vi "fpga_Ref Filter (60Hz).vi"(7 "reset":bool, 9 "input valid":bool, 11 "input data":fxp<+/-,24,1>) -> (1 "output valid":bool, 3 "output data <i24,3>":fxp<+/-,24,3> format="%.22g", 4 "ready for input":bool)   [LabVIEW 2011, in "NI_EP_Resample_FPGA.lvlib"]
uses:
  <vilib>/addons/Electrical Power/PQ/Resampling/NI_EP_Resample_FPGA.lvlib
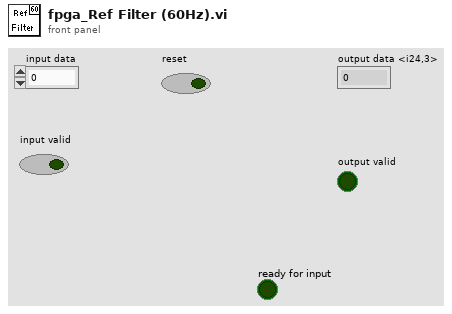
[diagram p1: front panel]
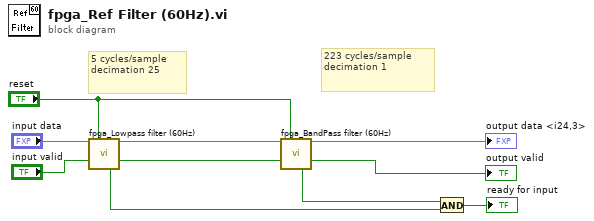
[diagram p0: block diagram]
diagram:
  # "223 cycles/sample\ndecimation 1"
  # "5 cycles/sample\ndecimation 25"
  n1 = call <vilib>:"fpga_Lowpass filter (60Hz).vi"("input data"="input data", "reset"="reset", "input valid"="input valid") -> ("output data"=w8:fxp<+/-,24,2>, "output valid"=w6:bool, "ready for input"=w2:bool)  [unwired: 10 in]
  n2 = call <vilib>:"fpga_BandPass filter (60Hz).vi"("input data"=w8, "reset"="reset", "input valid"=w6) -> ("output data"=→"output data <i24,3>":fxp<+/-,24,3>, "output valid"=→"output valid":bool, "ready for input"=w3:bool)  [unwired: 10 in]
  n3 = And(x=w3, y=w2) -> (x .and. y?=→"ready for input":bool)
